vi "Create Frame.vi"(8 "error in (no error)":errorcluster, 11 "Protocol Interface in":refnum<class "Protocol Interface.lvclass">) -> (0 "error out":errorcluster, 3 "Protocol Interface out":refnum<class "Protocol Interface.lvclass">)   [LabVIEW 2018]
uses:
  Protocol Interface.lvclass
  Protocol Type.ctl
panel:
  in  "Protocol Type":T1
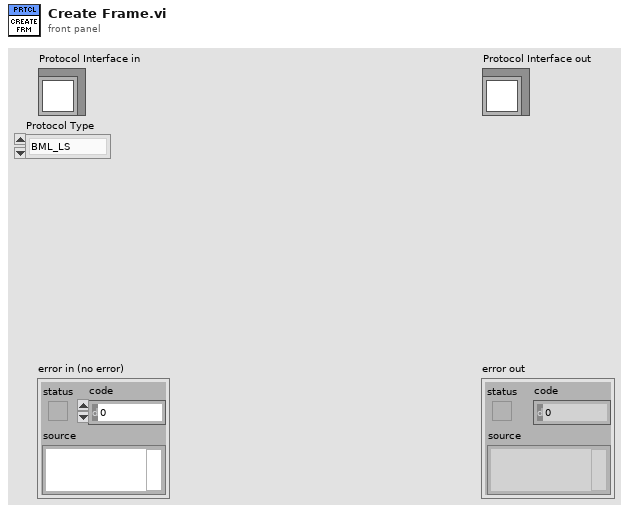
[diagram p1: front panel]
types:
  T1 = typedef "Protocol Interface.lvlib/Protocol Interface.lvclass/Protocol Type.ctl" = enum16{"BML_LS", "BML_HS", "SPI_3W", "SPI_4W"}
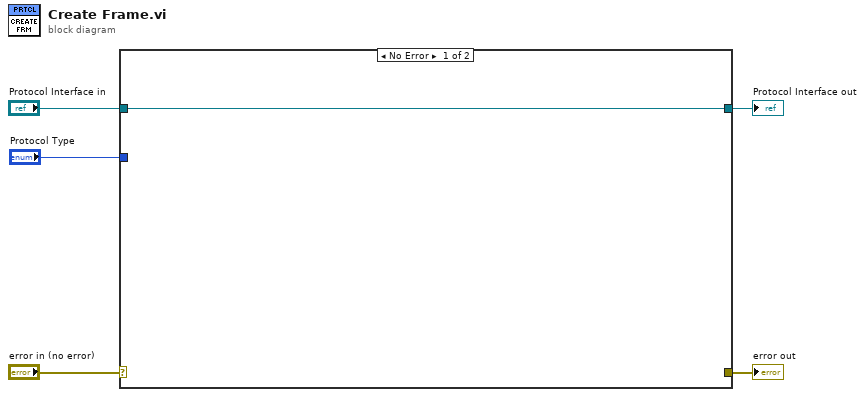
[diagram p0: block diagram]
diagram:
  n1 = case shown="No Error" "error in (no error)" {
    selector: "error in (no error)" -> [w8 w10]
    tunnel: [w7 w10] -> w4
    tunnel: [w6 w9] -> w2
    tunnel: "Protocol Interface in" -> [w6 w9]
    tunnel: "Protocol Type" -> [_ _]
    frame No Error {
    }
    frame Error {
    }
  }
  "error out" <- w4
  "Protocol Interface out" <- w2
